vi "check_is_moving.vi"(8 "error in (no error)":errorcluster, 11 "smc100 in":refnum<class "smc100.lvclass">) -> (0 "error out":errorcluster, 2 "Numeric":dbl, 3 "smc100 out":refnum<class "smc100.lvclass">)   [LabVIEW 2019, in "smc100.lvlib" / "smc100.lvclass"]
uses:
  smc100.lvclass
  smc100.lvclass/smc100.ctl
  Read VISA Handle.vi
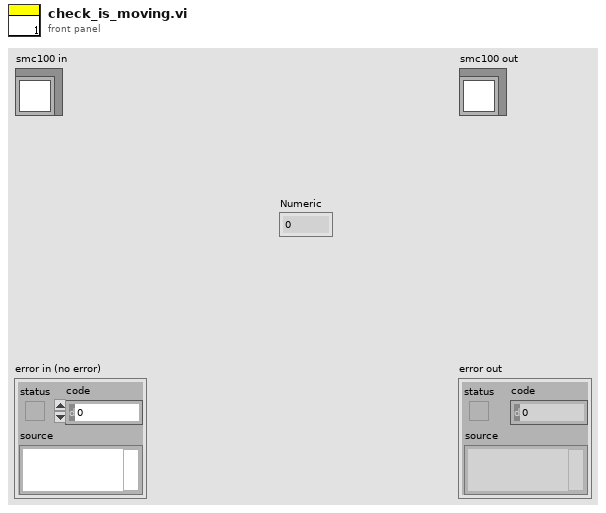
[diagram p1: front panel]
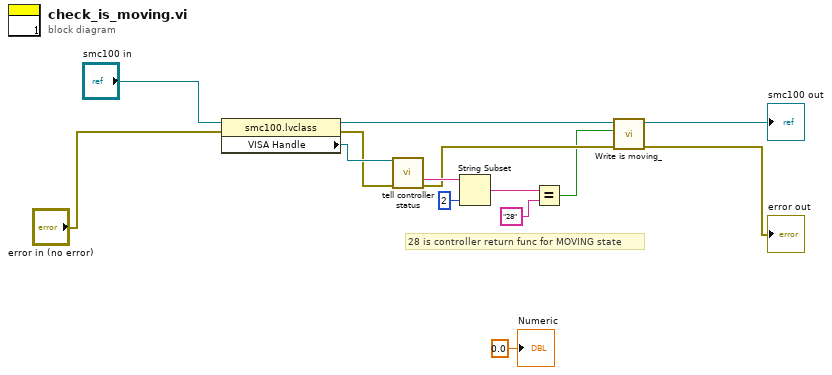
[diagram p0: block diagram]
diagram:
  # "28 is controller return func for MOVING state"
  n1 = property class="smc100.lvclass"(reference="smc100 in", error in="error in (no error)") -> (reference out=w6:refnum<class "smc100.lvclass">, error out=w12:errorcluster, "VISA Handle"=w13:refnum<visa-resource-name>)
  n2 = call <userlib>:"tell controller status.vi"("VISA Handle in"=w13, "error in"=w12) -> ("Controller's state"=w10:string, "error out"=w5:errorcluster)  [unwired: 8 in, 4 out]
  n3 = String Subset(string=w10, length (rest)=2 ("length (rest)")) -> (substring=w8:string)  [unwired: 1 in]
  n4 = Equal?(x=w8, y="28") -> (x = y?=w2:bool)
  n5 = call-dynamic "Write is moving_.vi"("error in (no error)"=w5, "is moving?"=w2, "_stage in"=w6) -> ("error out"=→"error out":errorcluster, "_stage out"=→"smc100 out":refnum<class "smc100.lvclass">)  [unwired: 7 in]
  "Numeric" <- 0.0 ("Numeric")
